vi "BotSpeak_DIORead.vi"(2 "Bot Settings":T1, 3 "DIO Line":u32) -> (1 "State":bool, 4 "Bot Settings out":T1)   [LabVIEW 2012]
doc: "Reads the value of the DIO pin specified by \"DIO Line\" and outputs the boolean \"State\" of the line."
uses:
  <userlib>/BotSpeak/VIs/Direct/BotSpeak_Control.ctl
panel:
  out "response":string
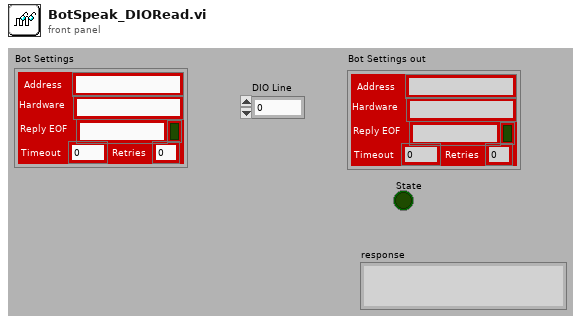
[diagram p1: front panel]
types:
  T1 = typedef "BotSpeak_Control.ctl" = cluster{"Address":string, "Reply EOF":string, "Hardware":string, "Retries":i8, "Timeout":i32, "Open?":bool}
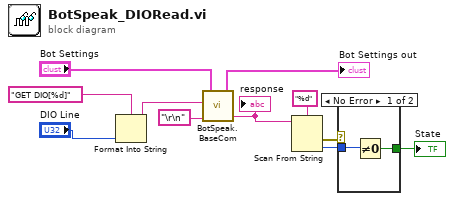
[diagram p0: block diagram]
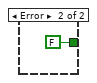
[diagram p2: hidden frame]
diagram:
  n1 = Format Into String(format string="GET DIO[%d]" ("command"), "DIO Line") -> (resulting string=w8:string)  [unwired: 2 in, 1 out]
  n2 = call <userlib>:"BotSpeak.BaseCom.vi"("Termination"="\r\n", "command"=w8, "Bot Settings in"="Bot Settings") -> ("response"=w1:string, "Bot Settings out"=→"Bot Settings out":T1)  [unwired: 2 in]
  "response" <- w1
  n3 = Scan From String(format string="%d", input string=w1) -> (error out=w2:errorcluster, output 1=w4:i32)  [unwired: 3 in, 2 out]
  n4 = case shown="No Error" w2 {
    tunnel: w4 -> [w13 _]
    tunnel: [w12 FALSE] -> w3
    frame No Error {
      n5 = Not Equal To 0?(x=w13) -> (x != 0?=w12:bool)
    }
    frame Error {
    }
  }
  "State" <- w3
